vi "VentiladorVI.vi"(8 "Aquisição pressão respiratória (cmH2O)":dbl, 9 "Pausa inspiração (s)":dbl=1.0, 10 "Limite pressão inspiratória (cmH2O)":dbl=2.0, 11 "Frequência respiratória (rpm)":dbl=6.0) -> (2 "Válvula expiração":dbl(graph), 3 "Válvula Inspiração":dbl(graph))   [LabVIEW 2019]
panel:
  in  "Incremento":dbl
  in  "Fluxo inicial":dbl
  in  "STOP":bool=TRUE
  out "Tempo do ciclo respiratório":u32(graph)
  in  "stop":bool
  in  "Tempo de respiração":dbl
  in  "Proporção Inspiração/respiração":string(combo)
  in  "Tipo de ventilação":string(combo)="Controlada"
  in  "Volume corrente":dbl
  in  "Tempo expiratório":dbl
  out "Fluxo respiratório medido":dbl
  in  "Fluxo respiratório set point":dbl
  # "rpm"
  # "(cmH2O)"
  # "(s)"
  # "\"Pausa inspiração\" neste programa está funcionando\ntambém como tempo de inspiração \ntotal, dado que não temos ainda nem \no controle nem a estimativa da rampa \nde subida da pressão do pulmão do paciente\npara diferenciar os valores"
  # "\"Vertical Pointer Slide\" está simulando a pressão\nno pulmão do paciente, você deve\n setá-lo para o valor de \"Limite pressão \ninspiratória\" quando Válvula inspiração =1 (aberta) e \nVálvula expiração = 0 (fechada) e para 0 (ou um valor \ndiferente de \"Limite pressão Inspiratória\") quando \nVálvula inspiração = 0 (fechada) e  Válvula expiração = 1 \n(aberta) para simular o ciclo de respiração natural."
  # "(s)"
  # "(s)"
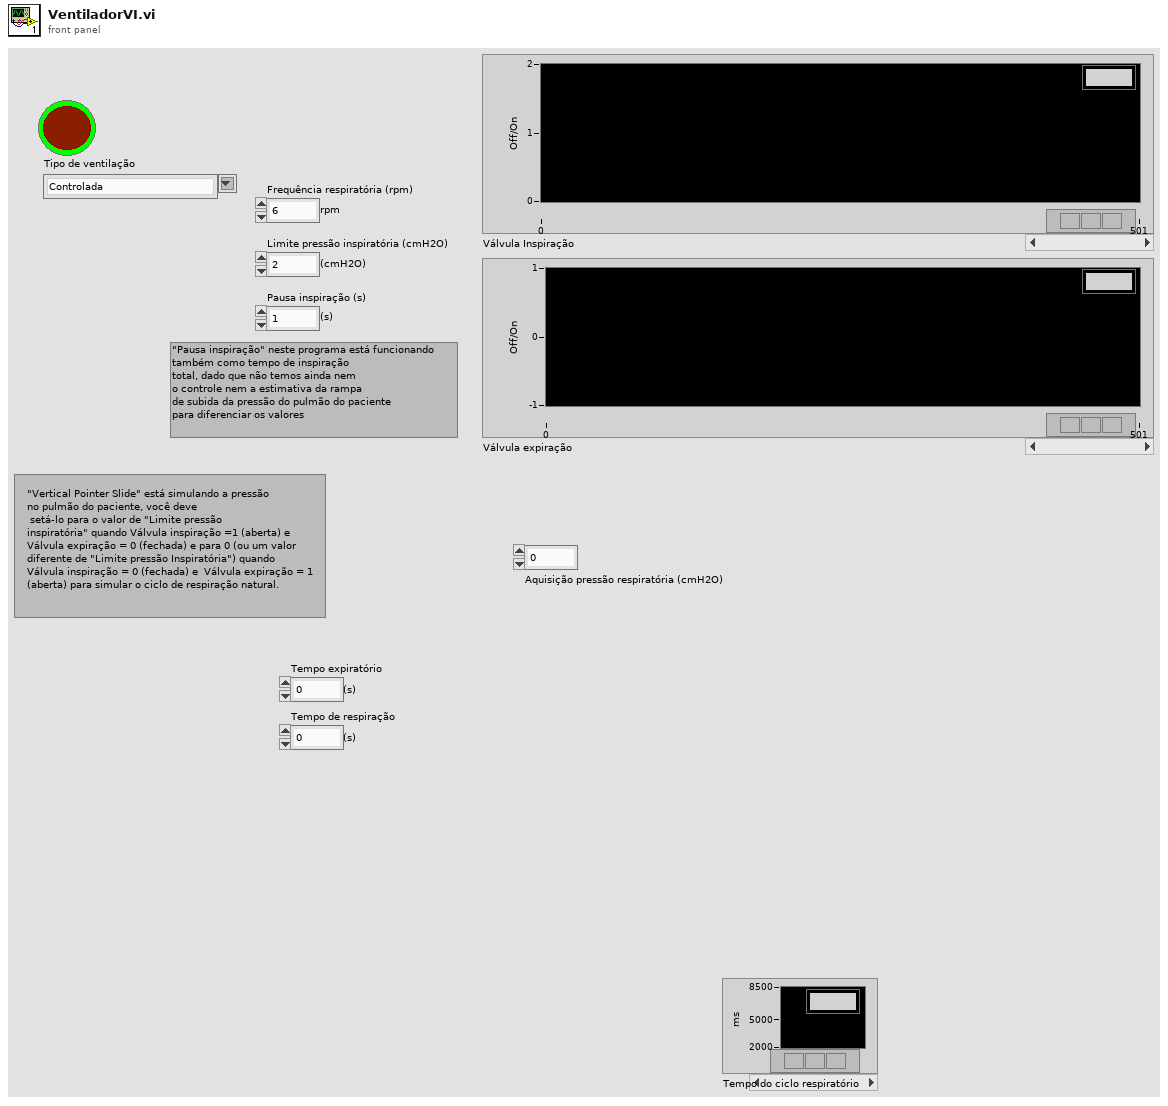
[diagram p1: front panel]
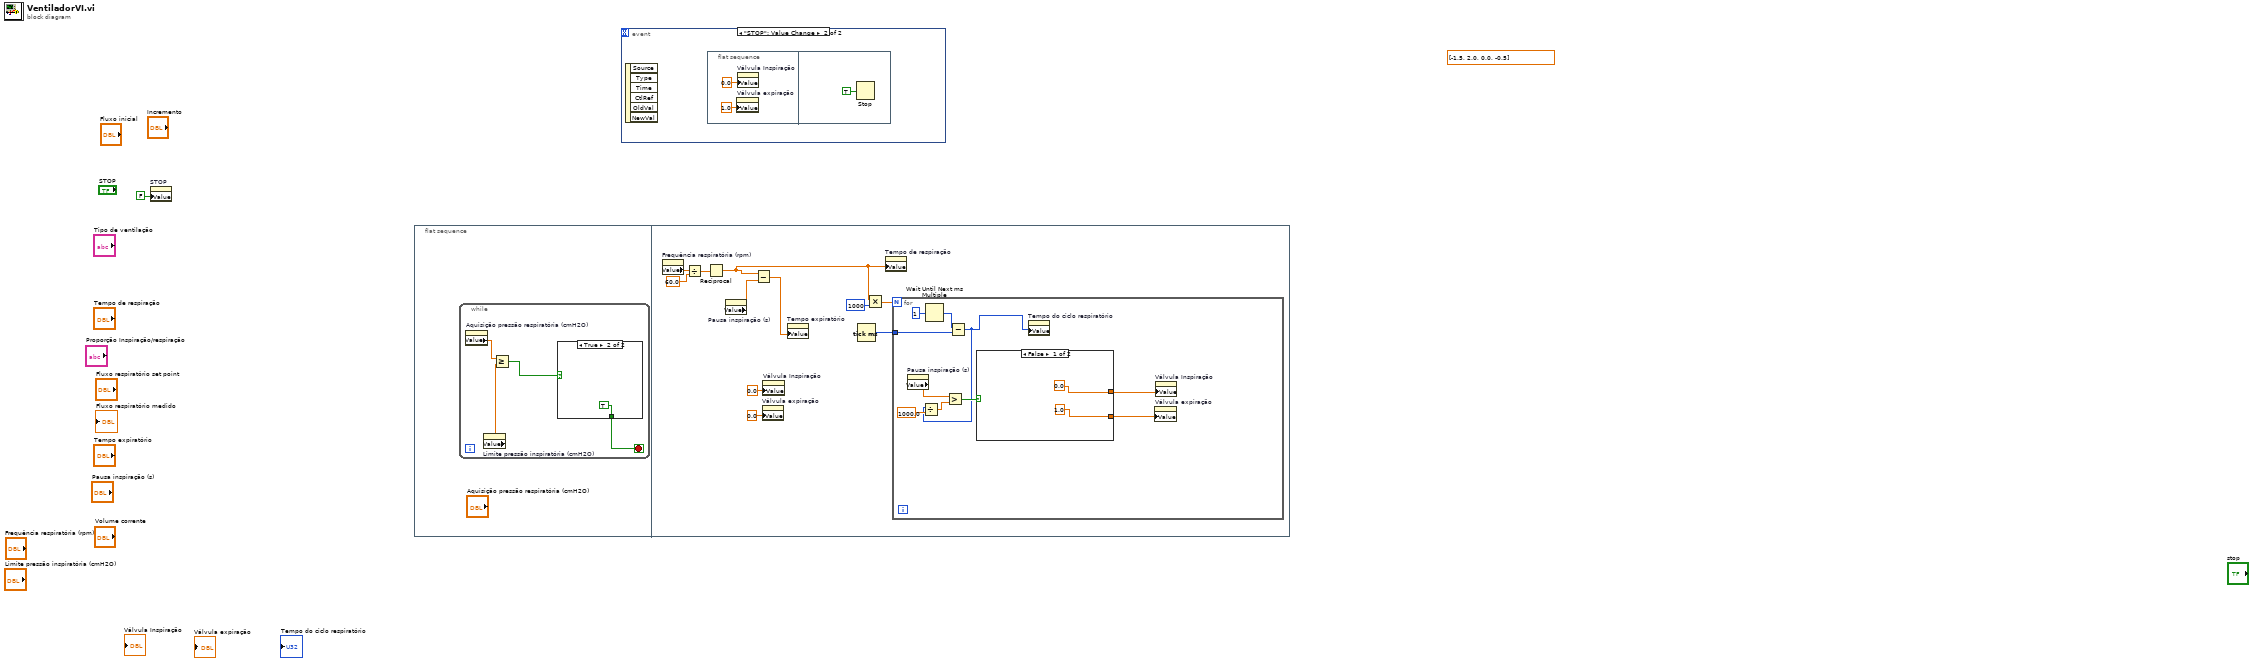
[diagram p0: block diagram]
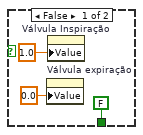
[diagram p2: hidden frame]
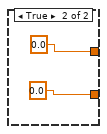
[diagram p3: hidden frame]
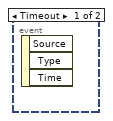
[diagram p4: hidden frame]
diagram:
  (unwired) dbl[] [-1.5, 2.0, 0.0, -0.5] ("P(x)")
  n1 = property on="STOP" class="Bool (strict)"("Value"=FALSE ("STOP")) -> ()  [unwired: 2 in, 2 out]
  n2 = flat-sequence {
    frame #0 {
      n3 = while {
        stop <- w2 stop-if-true
        n4 = property on="Aquisição pressão respiratória (cmH2O)" class="DigNum (strict)"() -> ("Value"=w3:dbl)  [unwired: 2 in, 2 out]
        n5 = property on="Limite pressão inspiratória (cmH2O)" class="DigNum (strict)"() -> ("Value"=w5:dbl)  [unwired: 2 in, 2 out]
        n6 = Greater Or Equal?(x=w3, y=w5) -> (x >= y?=w4:bool)
        n7 = case shown="True" w4 {
          tunnel: [FALSE TRUE] -> w2
          frame False {
            n8 = property on="Válvula expiração" class="WFChart (strict)"("Value"=0.0 ("Válvula expiração")) -> ()  [unwired: 2 in, 2 out]
            n9 = property on="Válvula Inspiração" class="WFChart (strict)"("Value"=1.0 ("Válvula Inspiração")) -> ()  [unwired: 2 in, 2 out]
          }
          frame True {
          }
        }
      }
    }
    frame #1 {
      n10 = property on="Frequência respiratória (rpm)" class="DigNum (strict)"() -> ("Value"=w17:dbl)  [unwired: 2 in, 2 out]
      n11 = Divide(x=w17, y=60.0) -> (x/y=w18:dbl)
      n12 = Reciprocal(x=w18) -> (1/x=w10:dbl)
      n13 = property on="Pausa inspiração (s)" class="DigNum (strict)"() -> ("Value"=w19:dbl)  [unwired: 2 in, 2 out]
      n14 = Subtract(x=w10, y=w19) -> (x-y=w20:dbl)
      n15 = property on="Válvula expiração" class="WFChart (strict)"("Value"=0.0 ("Válvula expiração")) -> ()  [unwired: 2 in, 2 out]
      n16 = property on="Válvula Inspiração" class="WFChart (strict)"("Value"=0.0 ("Válvula Inspiração")) -> ()  [unwired: 2 in, 2 out]
      n17 = property on="Tempo expiratório" class="DigNum (strict)"("Value"=w20) -> ()  [unwired: 2 in, 2 out]
      n18 = Tick Count (ms)() -> (millisecond timer value=w15:u32)
      n19 = Multiply(x=w10, y=1000) -> (x*y=w16:dbl)
      n20 = property on="Tempo de respiração" class="DigNum (strict)"("Value"=w10) -> ()  [unwired: 2 in, 2 out]
      n21 = for {
        N: w16 -> [_]
        tunnel: w15 -> [w28]
        n22 = property on="Pausa inspiração (s)" class="DigNum (strict)"() -> ("Value"=w26:dbl)  [unwired: 2 in, 2 out]
        n23 = Wait Until Next ms Multiple(millisecond multiple=u32 1) -> (millisecond timer value=w30:u32)
        n24 = Subtract(x=w30, y=w28) -> (x-y=w23:u32)
        n25 = Divide(x=w23, y=1000.0) -> (x/y=w25:dbl)
        n26 = Greater?(x=w26, y=w25) -> (0:w27:bool)
        n27 = case shown="False" w27 {
          tunnel: [0.0 ("Válvula Inspiração") 0.0 ("y")] -> w22
          tunnel: [1.0 ("Válvula expiração") 0.0 ("y")] -> w21
          frame False {
          }
          frame True {
          }
        }
        n28 = property on="Tempo do ciclo respiratório" class="WFChart (strict)"("Value"=w23) -> ()  [unwired: 2 in, 2 out]
        n29 = property on="Válvula expiração" class="WFChart (strict)"("Value"=w21) -> ()  [unwired: 2 in, 2 out]
        n30 = property on="Válvula Inspiração" class="WFChart (strict)"("Value"=w22) -> ()  [unwired: 2 in, 2 out]
      }
    }
  }
  n31 = event shown="[1] \"STOP\": Value Change" {
    selector: _ -> [_ _]
    dyn-events: _ -> [_ _]
    timeout: _ -> [_ _]
    event Timeout {
      n32 = event-data() -> ()  [unwired: 1 in, 3 out]
    }
    event "STOP": Value Change {
      n33 = event-data() -> ()  [unwired: 1 in, 6 out]
      n34 = flat-sequence {
        frame #0 {
          n35 = property on="Válvula expiração" class="WFChart (strict)"("Value"=1.0 ("Válvula expiração")) -> ()  [unwired: 2 in, 2 out]
          n36 = property on="Válvula Inspiração" class="WFChart (strict)"("Value"=0.0 ("Válvula Inspiração")) -> ()  [unwired: 2 in, 2 out]
        }
        frame #1 {
          n37 = Stop(stop? (T)=TRUE) -> ()
        }
      }
    }
  }
